vi "RateMatching.vi"(0 "PA":path, 1 "Nl":dbl, 2 "G":dbl, 3 "Nir":dbl, 5 "coded_data_DL":dbl[][](array[numeric]), 7 "Channel_type":dbl, 9 "error in (no error)":errorcluster caption="错误输入（无错误）", 11 "CpKpCmKmF":T1, 12 "direction":dbl, 13 "module_type":dbl, 14 "RVidx":dbl) -> (4 "rm_data":dbl[][](array[numeric]), 6 "rm_len":dbl[](array[numeric]), 10 "error out":errorcluster caption="错误输出")   [LabVIEW 2015]
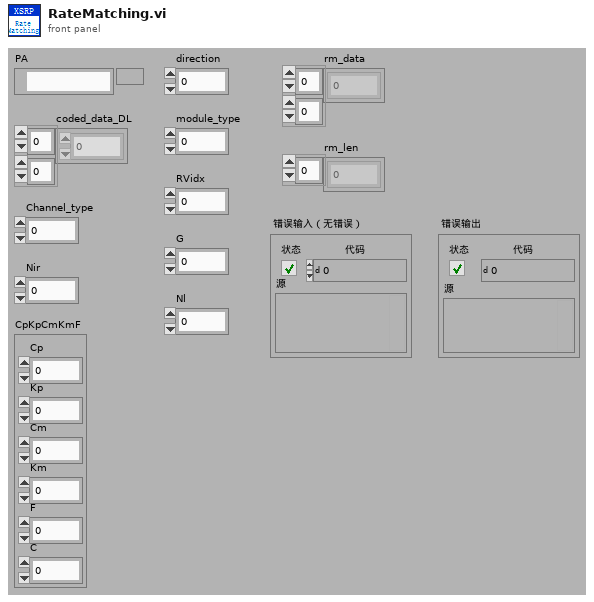
[diagram p1: front panel]
types:
  T1 = cluster{"Cp":dbl, "Kp":dbl, "Cm":dbl, "Km":dbl, "F":dbl, "C":dbl}
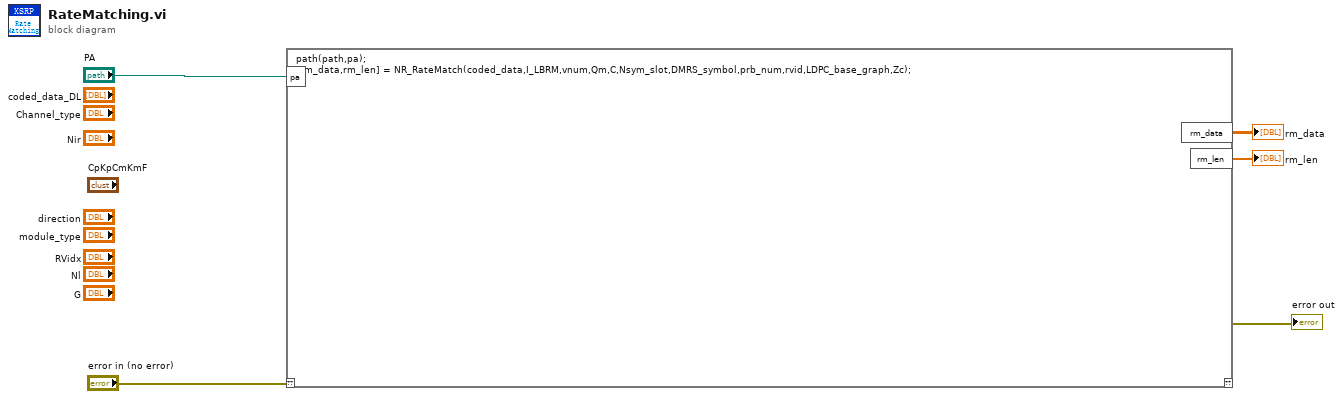
[diagram p0: block diagram]
diagram:
  n1 = script code="path(path,pa);\n[rm_data,rm_len] = NR_RateMatch(coded_data,I_LBRM,vnum,Qm,C,Nsym_slot,DMRS_symbol,prb_num,rvid,LDPC_base_graph,Zc);"("??"="error in (no error)", "pa"="PA") -> ("??"=→"error out":errorcluster, "rm_data"=→"rm_data":dbl[][], "rm_len"=→"rm_len":dbl[])
